vi "AddEventsLogToQ_Wrapper.vi"(8 "error in (no error)":errorcluster, 10 "spreadsheet string":string, 11 "EventType":string) -> (0 "error out":errorcluster)   [LabVIEW 2020]
uses:
  E84LoadPort/E84LoadPort.lvclass/E84LoadPort.ctl
  TD EventLogData--cluster.ctl
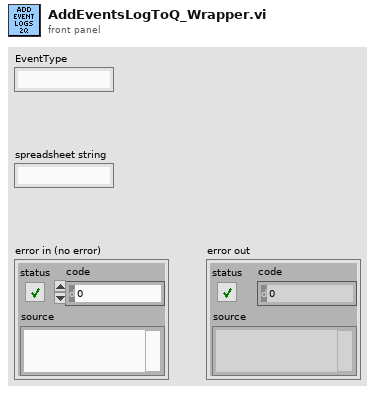
[diagram p1: front panel]
types:
  T1 = typedef "TD EventLogData--cluster.ctl" = cluster{"Timestamp":timestamp, "EventType":string, "EventData":string}
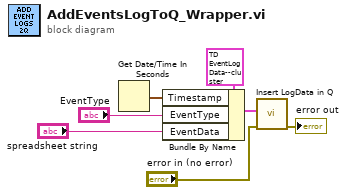
[diagram p0: block diagram]
diagram:
  n1 = Get Date/Time In Seconds() -> (seconds since 1Jan1904=w3:timestamp)
  n2 = Bundle By Name(cluster=T1 {"Timestamp"=timestamp(0 s since 1904-01-01), "EventType"="", "EventData"=""} ("EventLog"), "Timestamp"=w3, "EventType"="EventType", "EventData"="spreadsheet string") -> (w5:T1)
  n3 = call "Insert LogData in Q.vi"("error in (no error)"="error in (no error)", "EventLog"=w5) -> ("error out"=→"error out":errorcluster)  [unwired: 7 in, 2 out]
